vi "总磷总氮周期设置.vi"(11 "定时控制输入":T1={"控制命令"=enum."启动测量", "周期设置类型"=enum."定点启动", "定时功能启用"=FALSE, "定时间隔"=0.0, "24H周期设置"=[], "空白核查时间"=2, "跨度核查时间"=6, "质控频次"=enum."关闭"} {"跨度核查时间" items=["00H", "01H", "02H", "03H", "04H", "05H", "06H", "07H", "08H", "09H", "10H", "11H", "12H", "13H", "14H", "15H", "16H", "17H", "18H", "19H", "20H", "21H", "22H", "23H", "关闭"]; "空白核查时间" items=["00H", "01H", "02H", "03H", "04H", "05H", "06H", "07H", "08H", "09H", "10H", "11H", "12H", "13H", "14H", "15H", "16H", "17H", "18H", "19H", "20H", "21H", "22H", "23H", "关闭"]}) -> (3 "定时控制输出":T1={"控制命令"=enum."启动测量", "周期设置类型"=enum."定点启动", "定时功能启用"=FALSE, "定时间隔"=0.0, "24H周期设置"=[], "空白核查时间"=2, "跨度核查时间"=6, "质控频次"=enum."关闭"} {"跨度核查时间" items=["00H", "01H", "02H", "03H", "04H", "05H", "06H", "07H", "08H", "09H", "10H", "11H", "12H", "13H", "14H", "15H", "16H", "17H", "18H", "19H", "20H", "21H", "22H", "23H", "关闭"]; "空白核查时间" items=["00H", "01H", "02H", "03H", "04H", "05H", "06H", "07H", "08H", "09H", "10H", "11H", "12H", "13H", "14H", "15H", "16H", "17H", "18H", "19H", "20H", "21H", "22H", "23H", "关闭"]})   [LabVIEW 2016, in "斯坦道总磷.lvlib"]
uses:
  <vilib>/Utility/miscctls.llb/LVPointTypeDef.ctl
panel:
  in  "控制命令":T2(ring)
  in  "确定":bool
  in  "取消":bool
  in  "定时功能启用":bool
  out "选项卡控件":enum32{"定点启动", "间隔启动"}(tab)
  in  "质控频次":T3(ring)
  in  "跨度核查时间":u16(ring)=6 items=["00H", "01H", "02H", "03H", "04H", "05H", "06H", "07H", "08H", "09H", "10H", "11H", "12H", "13H", "14H", "15H", "16H", "17H", "18H", "19H", "20H", "21H", "22H", "23H", "关闭"]
  in  "空白核查时间":u16(ring)=2 items=["00H", "01H", "02H", "03H", "04H", "05H", "06H", "07H", "08H", "09H", "10H", "11H", "12H", "13H", "14H", "15H", "16H", "17H", "18H", "19H", "20H", "21H", "22H", "23H", "关闭"]
  in  "24H周期设置":bool[](xcontrol)
  in  "定时间隔":dbl
  in  "周期设置类型":enum16{"定点启动", "间隔启动"}(ring)
  # "仪器测试类型："
  # "周期设置类型："
  # "质控频次："
  # "零点核查时间："
  # "跨度核查时间："
  # "请输入定时启动间隔"
  # "min"
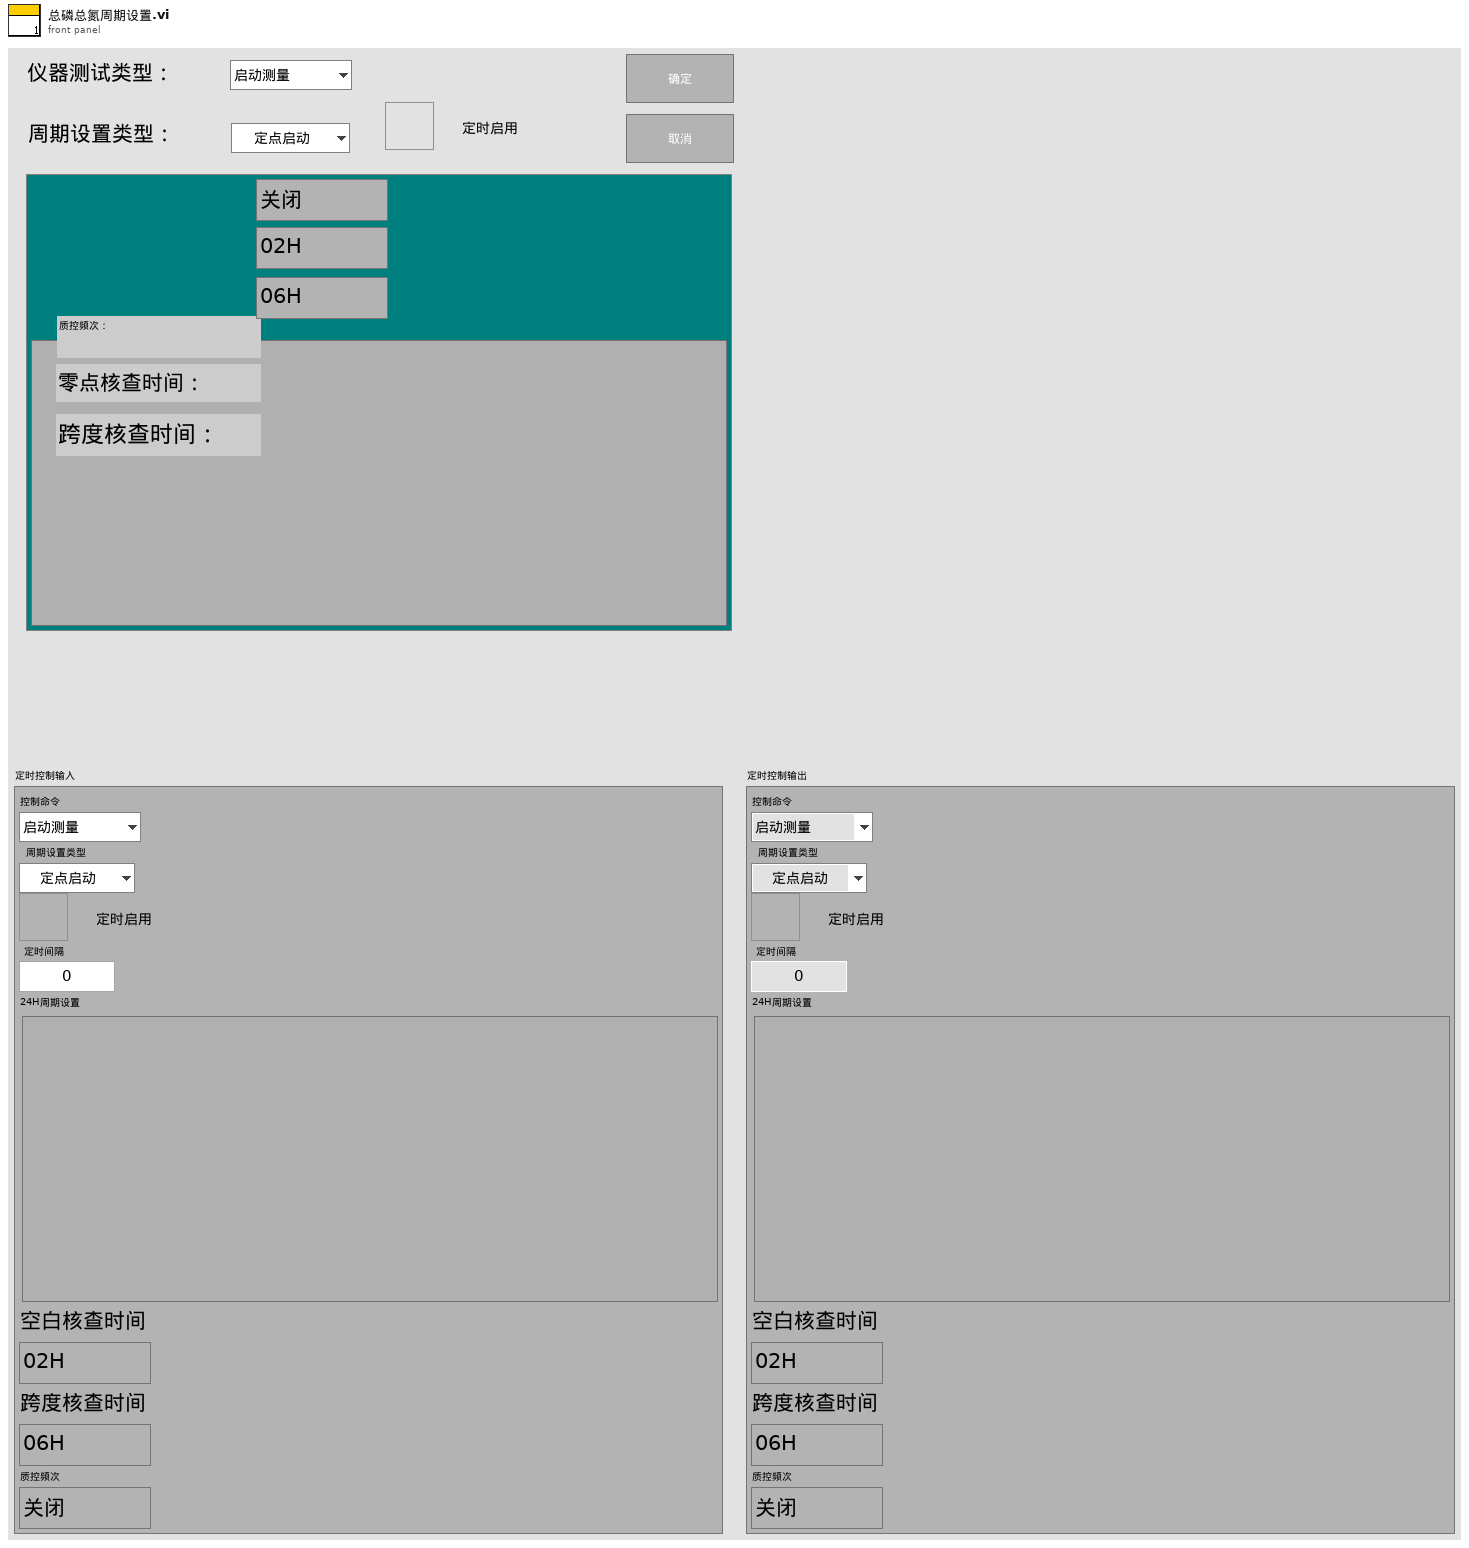
[diagram p1: front panel]
types:
  T1 = cluster{"控制命令":enum16{"启动测量", "标样核查", "零点核查", "跨度核查", "空白测试", "平行样测试", "加标回收", "空白校准", "标样校准", "初始化（清洗）", "停止测试", "仪器重启", "校时", "模式设置", "测量间隔设置"}, "周期设置类型":enum16{"定点启动", "间隔启动"}, "定时功能启用":bool, "定时间隔":dbl, "24H周期设置":bool[], "空白核查时间":u16, "跨度核查时间":u16, "质控频次":enum16{"关闭", "每天", "星期一", "星期二", "星期三", "星期四", "星期五", "星期六", "星期日"}}
  T2 = enum16{"启动测量", "标样核查", "零点核查", "跨度核查", "空白测试", "平行样测试", "加标回收", "空白校准", "标样校准", "初始化（清洗）", "停止测试", "仪器重启", "校时", "模式设置", "测量间隔设置"}
  T3 = enum16{"关闭", "每天", "星期一", "星期二", "星期三", "星期四", "星期五", "星期六", "星期日"}
  T4 = typedef "LVPointTypeDef.ctl" = cluster{"Horizontal":i16, "Vertical":i16}
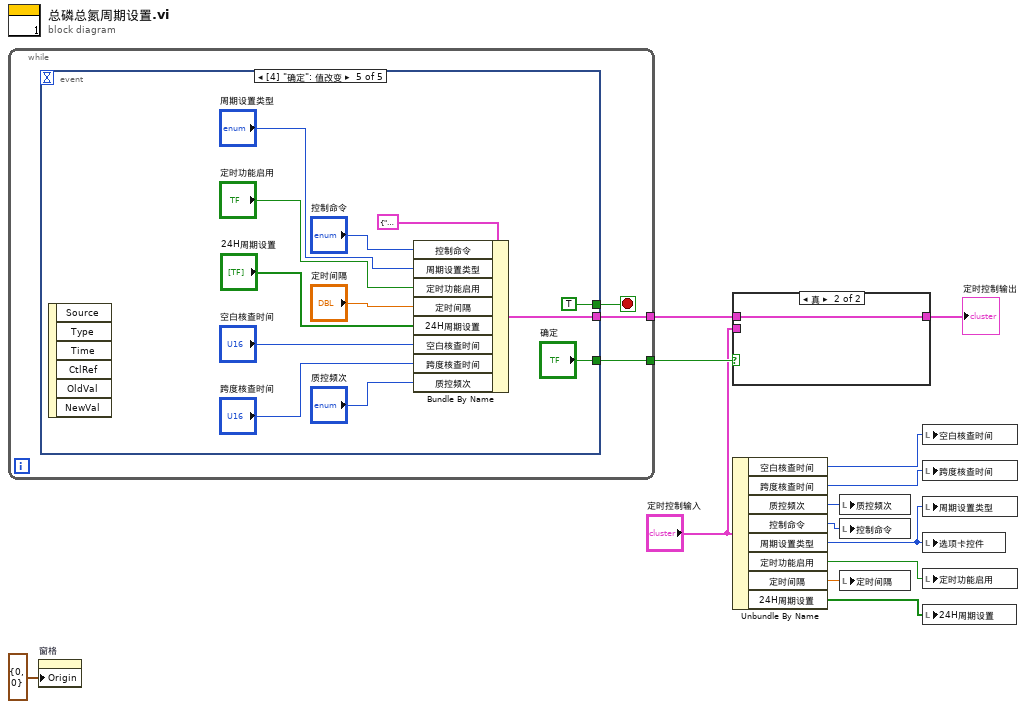
[diagram p0: block diagram]
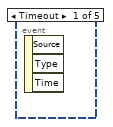
[diagram p3: hidden frame]
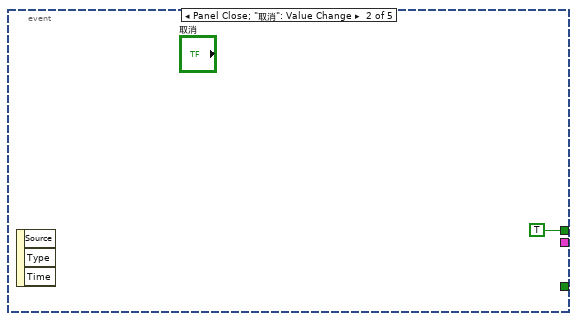
[diagram p4: hidden frame]
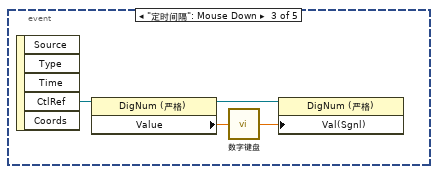
[diagram p5: hidden frame]
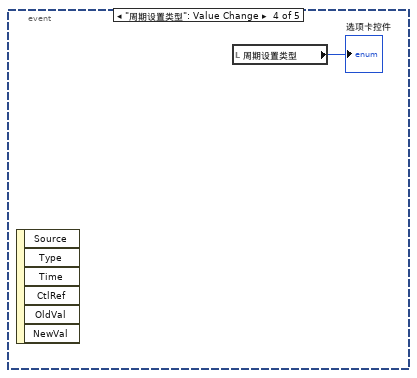
[diagram p6: hidden frame]
diagram:
  n1 = while {
    tunnel: [w15] -> w7
    tunnel: [w14] -> w8
    stop <- w16 stop-if-true
    n2 = event shown="[4] \"确定\": 值改变" {
      selector: _ -> [_ _ _ _ _]
      dyn-events: _ -> [_ _ _ _ _]
      timeout: _ -> [_ _ _ _ _]
      tunnel: [_ TRUE _ _ TRUE] -> w16
      tunnel: [_ _ _ _ w30] -> w15
      tunnel: [_ _ _ _ "确定"] -> w14
      event Timeout {
        n3 = event-data() -> ()  [unwired: 1 in, 3 out]
      }
      event Panel Close; "取消": Value Change {
        n4 = event-data() -> ()  [unwired: 1 in, 3 out]
      }
      event "定时间隔": Mouse Down {
        n5 = event-data() -> ("CtlRef"=w21:refnum<vi>)  [unwired: 1 in, 4 out]
        n6 = property class="DigNum (严格)"(reference=w21) -> (reference out=w18:refnum<vi>, "Value"=w20:dbl)  [unwired: 1 in, 1 out]
        n7 = call "数字键盘.vi"("OldNumber"=w20) -> ("NewNumber"=w19:dbl)
        n8 = property class="DigNum (严格)"(reference=w18, "Val(Sgnl)"=w19) -> ()  [unwired: 1 in, 2 out]
      }
      event "周期设置类型": Value Change {
        n9 = event-data() -> ()  [unwired: 1 in, 6 out]
        n10 = local read "周期设置类型"() -> (→"选项卡控件":enum16{"定点启动", "间隔启动"})
      }
      event "确定": Value Change {
        n11 = event-data() -> ()  [unwired: 1 in, 6 out]
        n12 = Bundle By Name(cluster=T1 {"控制命令"=enum."启动测量", "周期设置类型"=enum."定点启动", "定时功能启用"=FALSE, "定时间隔"=0.0, "24H周期设置"=[], "空白核查时间"=2, "跨度核查时间"=6, "质控频次"=enum."关闭"} ("定时控制输出"), "控制命令"="控制命令", "周期设置类型"="周期设置类型", "定时功能启用"="定时功能启用", "定时间隔"="定时间隔", "24H周期设置"="24H周期设置", "空白核查时间"="空白核查时间", "跨度核查时间"="跨度核查时间", "质控频次"="质控频次") -> (w30:T1)
      }
    }
  }
  n13 = property on="窗格" class="Pane"("Origin"=T4 {"Horizontal"=0, "Vertical"=0} ("原点")) -> ()  [unwired: 2 in, 2 out]
  n14 = case shown="真" w8 {
    tunnel: w7 -> [_ w36]
    tunnel: [w35 w36] -> w5
    tunnel: "定时控制输入" -> [w35 _]
    frame False {
    }
    frame True {
    }
  }
  "定时控制输出" <- w5
  n15 = Unbundle By Name("定时控制输入") -> ("空白核查时间"=w3:u16, "跨度核查时间"=w2:u16, "质控频次"=w1:T3, "控制命令"=w13:T2, "周期设置类型"=w9:enum16{"定点启动", "间隔启动"}, "定时功能启用"=w12:bool, "定时间隔"=w11:dbl, "24H周期设置"=w10:bool[])
  n16 = local write "质控频次"(w1) -> ()
  n17 = local write "控制命令"(w13) -> ()
  n18 = local write "定时间隔"(w11) -> ()
  n19 = local write "空白核查时间"(w3) -> ()
  n20 = local write "跨度核查时间"(w2) -> ()
  n21 = local write "周期设置类型"(w9) -> ()
  n22 = local write "选项卡控件"(w9) -> ()
  n23 = local write "定时功能启用"(w12) -> ()
  n24 = local write "24H周期设置"(w10) -> ()
